vi "CO2_switch_analysis.vi"() -> ()   [LabVIEW 2012]
uses:
  <vilib>/Analysis/3filter.llb/Filter Passband Type.ctl
  <vilib>/Utility/file.llb/Read From Spreadsheet File (DBL).vi
  <vilib>/Analysis/3filter.llb/Zero Phase Filter (DBL).vi
  <vilib>/Utility/file.llb/Write To Spreadsheet File (DBL).vi
  <vilib>/Analysis/NI_AALBase.lvlib
  <vilib>/gmath/NI_Gmath.lvlib
panel:
  out "XY Graph 5":cluster{"Value":dbl[], dbl[]}[](graph)
  in  "Gauss?":bool
  in  "Gauss width scale":dbl(slide) scale=0.0..5.0
  out "Pointer Frame":i32
  out "Point Time":dbl
  in  "Horizontal plot range 3":i32(slide)=564 scale=415.36414565826334..795.514205682273
  out "Analysis Time":dbl
  in  "Multiply SD in Lock-in?":bool
  in  "Average Window":i32(slide)=20 scale=0.0..20.0
  in  "Horizontal plot range 2":cluster{i32, i32, i32, dbl}(slide)={529, 548, 526, 593.2768414505381} scale=403.8640519766044..784.014195885828
  in  "Square Lock-in?":bool
  out "XY Graph 4":cluster{"all rows":dbl[], "all rows":dbl[]}[](graph)
  in  "Lock-in phase":dbl(slide)=2.317171717171717 scale=0.0..6.2
  in  "Lock-in sine Period":dbl(slide)=20.0 step=0.001 scale=19.9..20.1
  out "XY Graph 3":cluster{"Value":dbl[], "Value":dbl[]}[](graph)
  in  "High Pass Filter?":bool=TRUE
  out "1/x":dbl=0.4001580462202354
  in  "Filter order":i32=2
  in  "lowpass":dbl(slide)=0.01 scale=0.0..0.02
  out "Output":dbl[][](array[numeric])
  in  "Write Data":bool
  out "ESCRT":dbl[](array[numeric])
  in  "Horizontal plot range":cluster{i32, i32}(slide)={1038, 1988} scale=0.0..4250.0
  in  "Window":i32(slide)=24 scale=0.0..100.0
  in  "Plot":bool
  in  "Load Data":bool
  out "Data":dbl[][](array[numeric]) format="%0.3f"
  in  "file path (dialog if empty)":path
  in  "stop":bool=TRUE
  out "XY Graph 2":cluster{"Value":dbl[], "Value":dbl[]}[](graph)
  out "XY Graph":cluster{"all rows":dbl[], "all rows":dbl[]}[](graph)
  in  "ESCRT amplitude":i32=22
  in  "Gag Amplitude":i32=12
  in  "Time":i32=3
  out "Time":dbl[](array[numeric])
  # "This program is used to analyze CO2 dependent oscilaltions to determine scission moment. Puncta amplitudes are input as spreedsheet and filtered\nwith lock-in technique using reference that is same frequency as CO2 modulation frequency. The lock-in signal is used to determine scission time. \nTiming of ESCRT recruitment is also determined from amplitude of ESCRT signal."
  # "Array Index"
  # "Column 22. ESCRT Avg Intensity"
  # "Column 23. ESCRT Intensity SD"
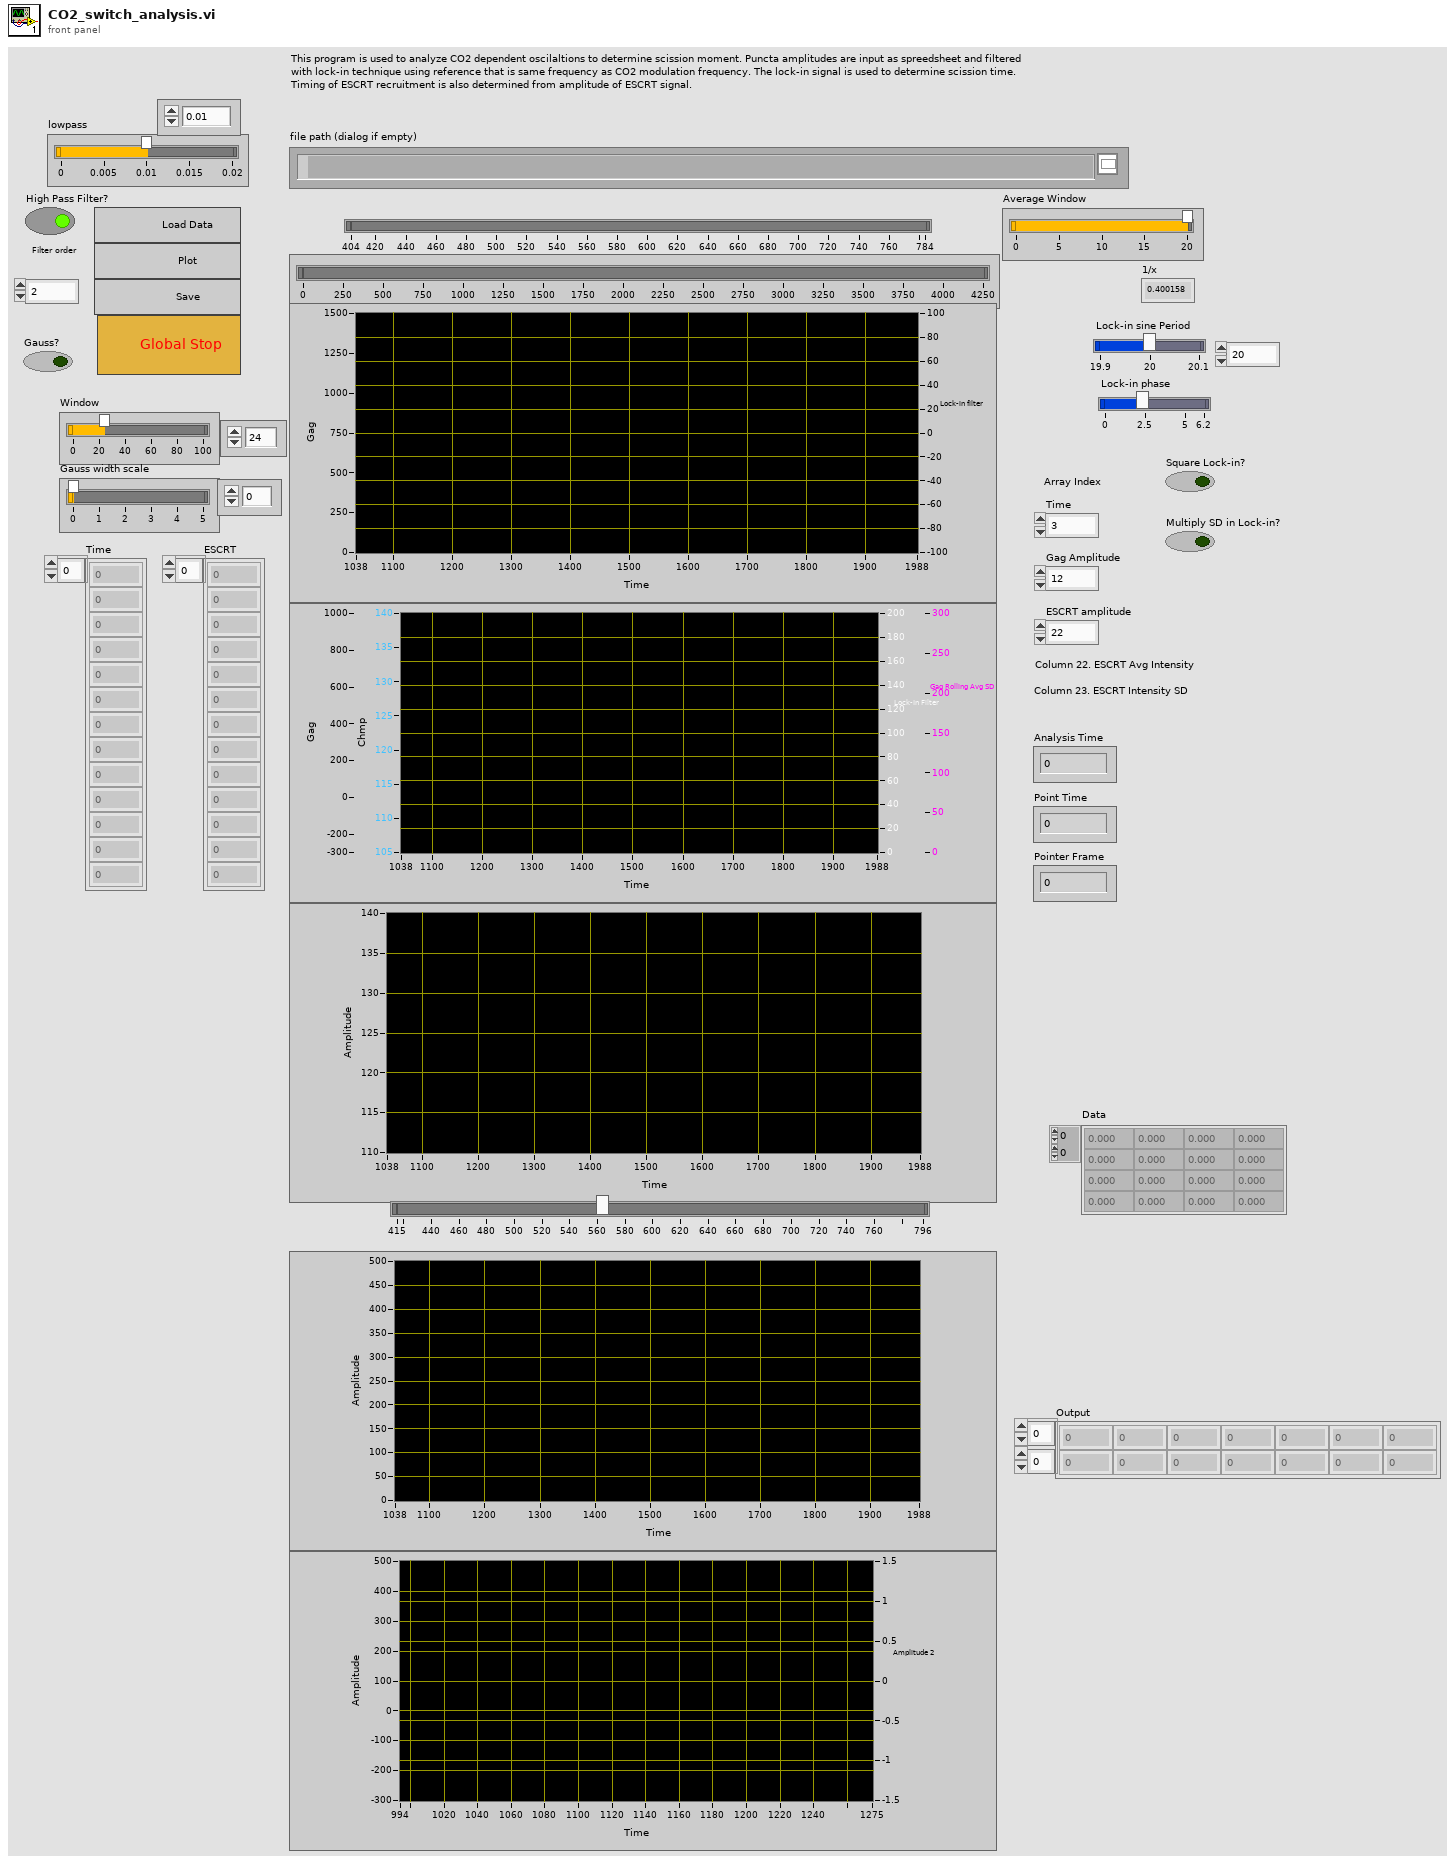
[diagram p1: front panel]
types:
  T1 = typedef "NI_AALBase.lvlib/Filter Passband Type.ctl" = enum32{"Lowpass", "Highpass", "Bandpass", "Bandstop"}
  T2 = cluster{"filter structure":enum32{"IIR 2nd Order", "IIR 4th Order"}, "Reverse Coefficients":dbl[], "Forward Coefficients":dbl[]}
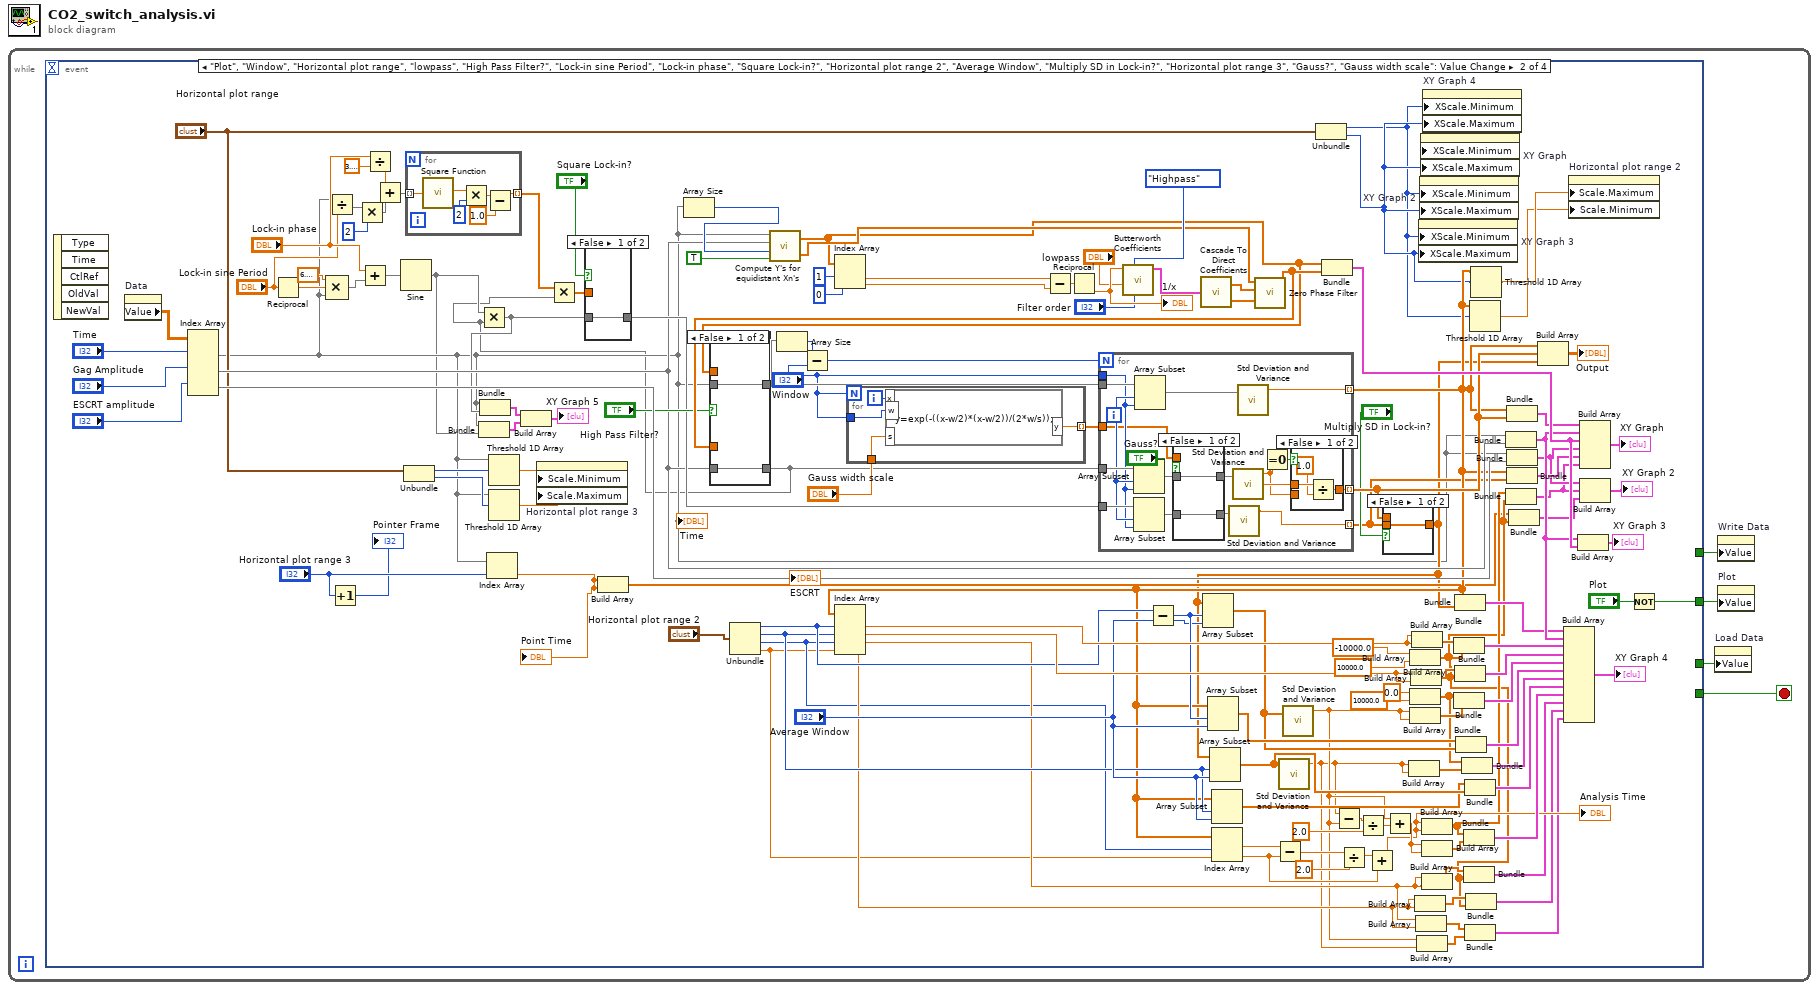
[diagram p0: block diagram]
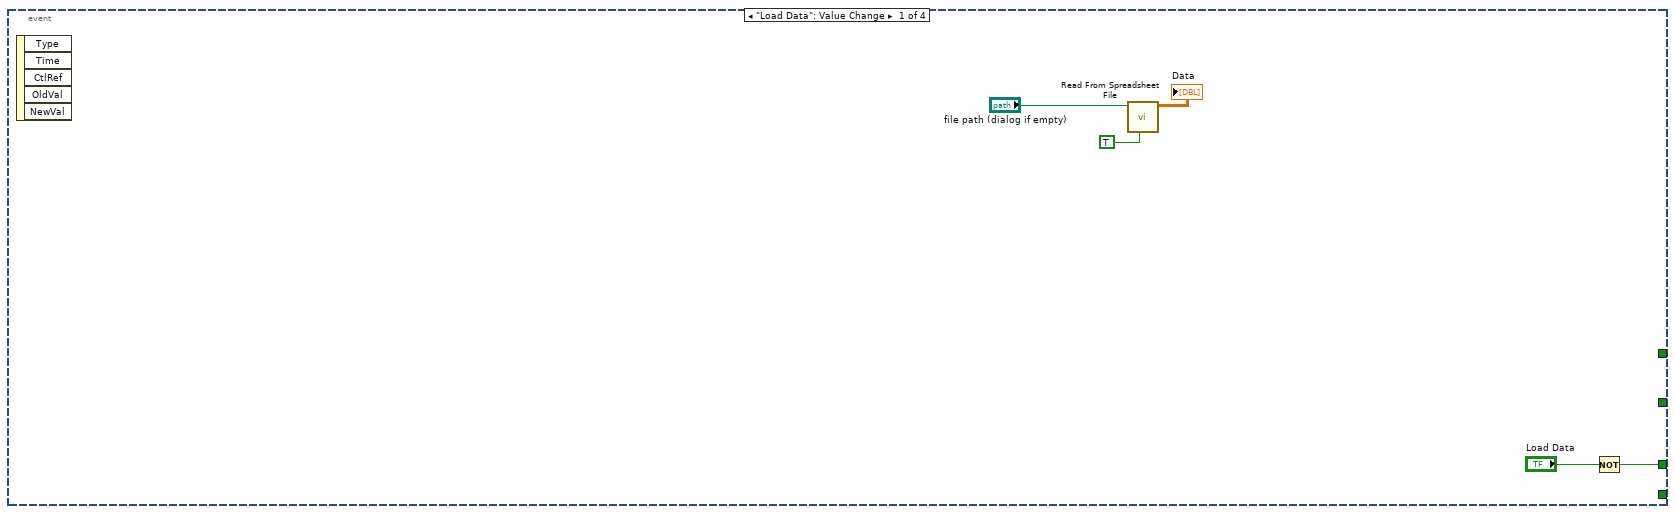
[diagram p2: hidden frame]
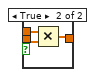
[diagram p3: hidden frame]
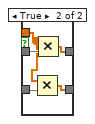
[diagram p6: hidden frame]
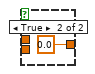
[diagram p7: hidden frame]
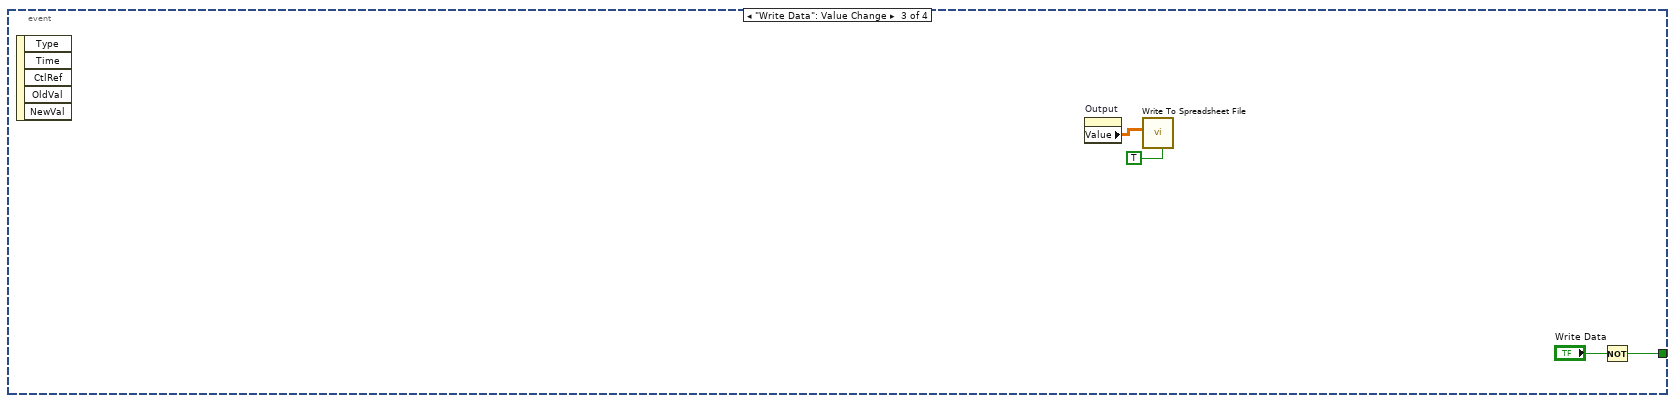
[diagram p8: hidden frame]
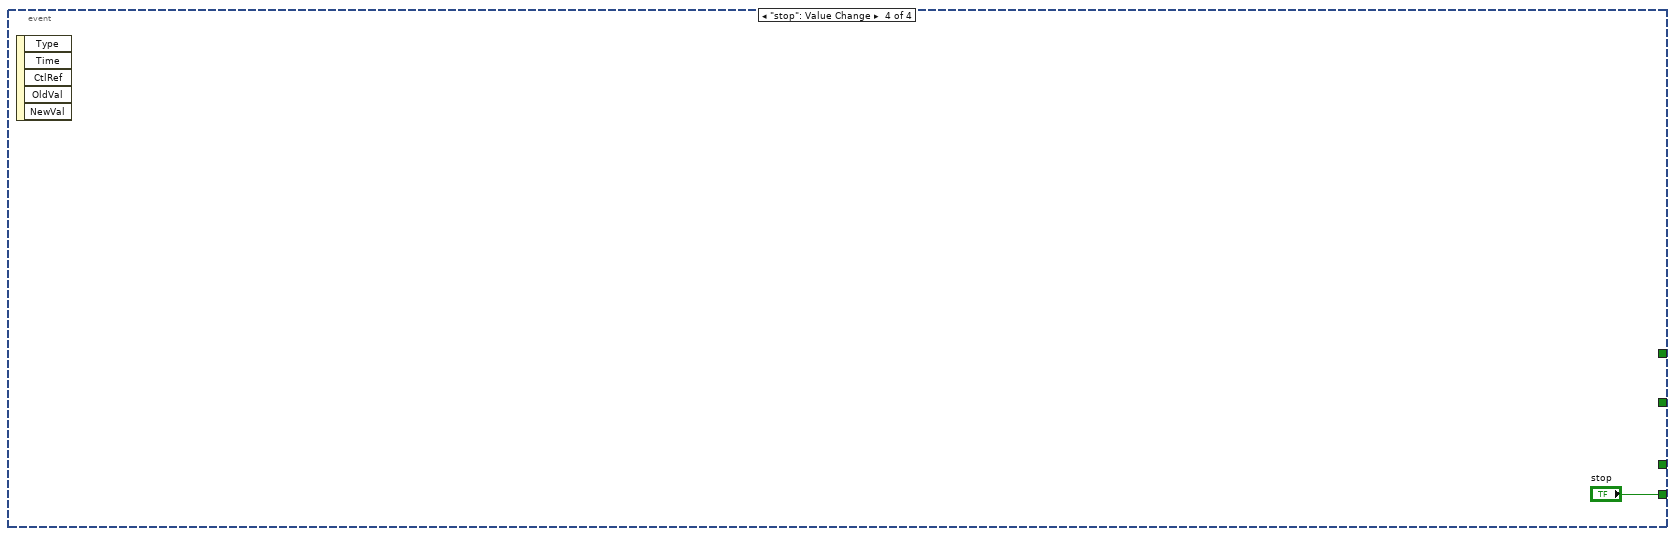
[diagram p9: hidden frame]
diagram:
  n1 = while {
    stop <- w4 stop-if-true
    n2 = event shown="[1] \"Plot\", \"Window\", \"Horizontal plot range\", \"lowpass\", \"High Pass Filter?\", \"Lock-in sine Period\", \"Lock-in phase\", \"Square Lock-in?\", \"Horizontal plot range 2\", \"Average Window\", \"Multiply SD in Lock-in?\", \"Horizontal plot range 3\", \"Gauss?\", \"Gauss width scale\": Value Change" {
      selector: _ -> [_ _ _ _]
      dyn-events: _ -> [_ _ _ _]
      timeout: _ -> [_ _ _ _]
      tunnel: [_ _ _ "stop"] -> w4
      tunnel: [w5 _ _ _] -> w3
      tunnel: [_ w147 _ _] -> w2
      tunnel: [_ _ w200 _] -> w1
      event "Load Data": Value Change {
        n3 = event-data() -> ()  [unwired: 1 in, 5 out]
        n4 = call-poly <vilib>:"Read From Spreadsheet File.vi"("transpose (no:F)"=TRUE, "file path (dialog if empty)"="file path (dialog if empty)") -> ("all rows"=→"Data":dbl[][])  [unwired: 5 in, 4 out]
        n5 = Not(x="Load Data") -> (.not. x?=w5:bool)
      }
      event "Plot", "Window", "Horizontal plot range", "lowpass", "High Pass Filter?", "Lock-in sine Period", "Lock-in phase", "Square Lock-in?", "Horizontal plot range 2", "Average Window", "Multiply SD in Lock-in?", "Horizontal plot range 3", "Gauss?", "Gauss width scale": Value Change {
        n6 = event-data() -> ()  [unwired: 1 in, 5 out]
        n7 = property on="Data" class="Arr (strict)"() -> ("Value"=w142:dbl[][])  [unwired: 2 in, 2 out]
        n8 = Index Array(array=w142, index (row) #1="Time", index (row) #2="Gag Amplitude", index (row) #3="ESCRT amplitude") -> (element #1=w15:dbl[], element #2=w90:dbl[], element #3=w141:dbl[])  [unwired: 3 in]
        "Time" <- w15
        "ESCRT" <- w141
        n9 = Reciprocal(x="Lock-in sine Period") -> (1/x=w116:dbl)
        n10 = Compound Arithmetic op=MULTIPLY(6.283185307179586, w116, w15) -> (w115:dbl[])
        n11 = Divide(x=w15, y="Lock-in sine Period") -> (x/y=w100:dbl[])
        n12 = Increment(x="Horizontal plot range 3") -> (x+1=→"Pointer Frame":i32)
        n13 = Multiply(x=w100, y=2) -> (x*y=w98:dbl[])
        n14 = Add(x="Lock-in phase", y=w115) -> (x+y=w114:dbl[])
        n15 = Divide(x="Lock-in phase", y=3.141592653589793) -> (x/y=w107:dbl)
        n16 = Add(x=w107, y=w98) -> (x+y=w106:dbl[])
        n17 = Sine(x=w114) -> (sin(x)=w14:dbl[])
        n18 = Unbundle("Horizontal plot range") -> (w30:i32, w29:i32)
        n19 = for {
          tunnel: w106 -> [w164] mode=indexing
          tunnel: [w160] -> w102 mode=indexing
          n20 = call <vilib>:"Square Function.vi"("x"=w164) -> ("square(x)"=w163:dbl)
          n21 = Multiply(x=w163, y=2) -> (x*y=w161:dbl)
          n22 = Subtract(x=w161, y=1.0) -> (x-y=w160:dbl)
        }
        n23 = Bundle("Value"=w15, w14) -> (w12:cluster{"Value":dbl[], dbl[]})  [unwired: 1 in]
        n24 = Index Array(array=w15, index="Horizontal plot range 3") -> (element=w31:dbl)
        "Point Time" <- w31
        n25 = Threshold 1D Array(2:w30, 3:w15) -> (0:w25:dbl)  [unwired: 1 in]
        n26 = Threshold 1D Array(2:w29, 3:w15) -> (0:w24:dbl)  [unwired: 1 in]
        n27 = property on="Horizontal plot range 3" class="Slide (strict)"("Scale.Minimum"=w25, "Scale.Maximum"=w24) -> ()  [unwired: 2 in, 2 out]
        n28 = Build Array(w31, w31) -> (w32:dbl[])
        n29 = Array Size(array=w15) -> (size(s)=w120:i32)
        n30 = Unbundle("Horizontal plot range 2") -> (w73:i32, w72:i32, w39:i32, w38:dbl)
        n31 = call "Compute Y's for equidistant Xn's.vi"("Spline(T)"=TRUE, "N"=w120, "Y"=w90, "X"=w15) -> ("Yequi"=w126:dbl[], "Xequi"=w124:dbl[])
        n32 = Index Array(array=w124, index #1=1 ("index"), index #2=0 ("index")) -> (element #1=w136:dbl, element #2=w135:dbl)
        n33 = for {
          N: "Window" -> [_]
          tunnel: "Window" -> [w151]
          tunnel: "Gauss width scale" -> [w150]
          tunnel: [w149] -> w18 mode=indexing
          i -> [w152]
          n34 = formula code="y=exp(-((x-w/2)*(x-w/2))/(2*w/s));"("x"=w152, "w"=w151, "s"=w150) -> ("y"=w149:dbl)
        }
        n35 = Subtract(x=w136, y=w135) -> (x-y=w134:dbl)
        n36 = Reciprocal(x=w134) -> (1/x=w133:dbl)
        "1/x" <- w133
        n37 = call <vilib>:"Butterworth Coefficients.vi"("order"="Filter order", "filter type"=Filter_Passband_Type."Highpass", "low cutoff freq: fl"="lowpass", "sampling freq: fs"=w133) -> ("IIR Filter Cluster"=w129:T2)  [unwired: 6 in, 1 out]
        n38 = Subtract(x=w73, y="Average Window") -> (x-y=w84:i32)
        n39 = call <vilib>:"Cascade To Direct Coefficients.vi"("IIR Filter Cluster"=w129) -> ("Reverse Coefficients"=w128:dbl[], "Forward Coefficients"=w127:dbl[])
        n40 = call-poly <vilib>:"Zero Phase Filter.vi"("Forward Coefficients"=w127, "Reverse Coefficients"=w128, "X"=w126) -> ("Filtered X"=w125:dbl[])  [unwired: 7 in, 1 out]
        n41 = case shown="False" "High Pass Filter?" {
          tunnel: [w166 w168] -> w10
          tunnel: w90 -> [w166 _]
          tunnel: [w165 w167] -> w122
          tunnel: w15 -> [w165 _]
          tunnel: w125 -> [_ w168]
          tunnel: w124 -> [_ w167]
          frame False {
          }
          frame True {
          }
        }
        n42 = Multiply(x=w14, y=w10) -> (x*y=w16:dbl[])
        n43 = Bundle("Value"=w15, w16) -> (w13:cluster{"Value":dbl[], dbl[]})  [unwired: 1 in]
        n44 = Build Array(w13, w12) -> (→"XY Graph 5":cluster{"Value":dbl[], dbl[]}[])
        n45 = Multiply(x=w102, y=w10) -> (x*y=w105:dbl[])
        n46 = case shown="False" "Square Lock-in?" {
          tunnel: w16 -> [w157 _]
          tunnel: [w157 w158] -> w103
          tunnel: w105 -> [_ w158]
          frame False {
          }
          frame True {
          }
        }
        n47 = Array Size(array=w122) -> (size(s)=w123:i32)
        n48 = Subtract(x=w123, y="Window") -> (x-y=w20:i32)
        n49 = for {
          N: w20 -> [_]
          tunnel: w122 -> [w186]
          tunnel: "Window" -> [w176]
          tunnel: [w184] -> w59 mode=indexing
          tunnel: w10 -> [w183]
          tunnel: [w180] -> w61 mode=indexing
          tunnel: [w169] -> w58 mode=indexing
          tunnel: w103 -> [w178]
          tunnel: w18 -> [w173]
          i -> [w177]
          n50 = Array Subset(array=w183, index=w177, length=w176) -> (w175:dbl[])
          n51 = Array Subset(array=w178, index=w177, length=w176) -> (w171:dbl[])
          n52 = Array Subset(array=w186, index=w177, length=w176) -> (w185:dbl[])
          n53 = case shown="False" "Gauss?" {
            tunnel: w175 -> [w188 w193]
            tunnel: [w188 w192] -> w174
            tunnel: w173 -> [_ w189]
            tunnel: w171 -> [w187 w190]
            tunnel: [w187 w191] -> w170
            frame False {
            }
            frame True {
              n54 = Multiply(x=w189, y=w190) -> (x*y=w191:dbl[])
              n55 = Multiply(x=w189, y=w193) -> (x*y=w192:dbl[])
            }
          }
          n56 = call <vilib>:"Std Deviation and Variance.vi"("X"=w170) -> ("mean"=w169:dbl)  [unwired: 1 in, 2 out]
          n57 = call <vilib>:"Std Deviation and Variance.vi"("X"=w174) -> ("mean"=w179:dbl, "standard deviation"=w181:dbl)  [unwired: 1 in, 1 out]
          n58 = call <vilib>:"Std Deviation and Variance.vi"("X"=w185) -> ("mean"=w184:dbl)  [unwired: 1 in, 2 out]
          n59 = Equal To 0?(x=w179) -> (x = 0?=w182:bool)
          n60 = case shown="False" w182 {
            tunnel: w179 -> [_ _]
            tunnel: w181 -> [w196 _]
            tunnel: [w195 0.0] -> w180
            frame False {
              n61 = Divide(x=w196, y=1.0) -> (x/y=w195:dbl)
            }
            frame True {
            }
          }
        }
        n62 = Index Array(array=w59, index #1=w73, index #2=w72, index #3=w39, index #4=w38) -> (element #1=w89:dbl, element #2=w93:dbl, element #3=w47:dbl, element #4=w46:dbl)
        n63 = Array Subset(array=w59, index=w84, length="Average Window") -> (w83:dbl[])
        n64 = Array Subset(array=w59, index=w72, length="Average Window") -> (w76:dbl[])
        n65 = Index Array(array=w59, index #1=w39, index #2=w38) -> (element #1=w66:dbl, element #2=w62:dbl)
        n66 = Subtract(x=w66, y=w62) -> (x-y=w65:dbl)
        n67 = Unbundle("Horizontal plot range") -> (w35:i32, w36:i32)
        n68 = Bundle("Xequi"=w124, "Filtered X"=w125) -> (w118:cluster{"Xequi":dbl[], "Filtered X":dbl[]})  [unwired: 1 in]
        n69 = Divide(x=w65, y=2.0) -> (x/y=w63:dbl)
        n70 = Add(x=w63, y=w62) -> (x+y=w56:dbl)
        "Analysis Time" <- w56
        n71 = case shown="False" "Multiply SD in Lock-in?" {
          tunnel: w58 -> [w153 w155]
          tunnel: [w153 w156] -> w21
          tunnel: w61 -> [_ w154]
          frame False {
          }
          frame True {
            n72 = Multiply(x=w154, y=w155) -> (x*y=w156:dbl[])
          }
        }
        n73 = Array Subset(array=w21, index=w84, length="Average Window") -> (w82:dbl[])
        n74 = Array Subset(array=w21, index=w72, length="Average Window") -> (w77:dbl[])
        n75 = call <vilib>:"Std Deviation and Variance.vi"("X"=w77) -> ("mean"=w44:dbl)  [unwired: 1 in, 2 out]
        n76 = call <vilib>:"Std Deviation and Variance.vi"("X"=w82) -> ("mean"=w45:dbl)  [unwired: 1 in, 2 out]
        n77 = Subtract(x=w44, y=w45) -> (x-y=w70:dbl)
        n78 = Divide(x=w70, y=2.0) -> (x/y=w68:dbl)
        n79 = Add(x=w45, y=w68) -> (x+y=w67:dbl)
        n80 = Build Array(w44, w44) -> (w79:dbl[])
        n81 = Build Array(-10000.0 ("element"), 10000.0 ("element")) -> (w33:dbl[])
        n82 = Build Array(0.0 ("element"), 10000.0 ("element")) -> (w80:dbl[])
        n83 = Build Array(w45, w45) -> (w86:dbl[])
        n84 = Build Array(w93, w93) -> (w92:dbl[])
        n85 = Build Array(w89, w89) -> (w96:dbl[])
        n86 = Build Array(w46, w46) -> (w49:dbl[])
        n87 = Build Array(w47, w46) -> (w42:dbl[])
        n88 = Build Array(w45, w44) -> (w43:dbl[])
        n89 = property on="XY Graph 3" class="XYGraph (strict)"("XScale.Minimum"=w35, "XScale.Maximum"=w36) -> ()  [unwired: 2 in, 2 out]
        n90 = property on="XY Graph 2" class="XYGraph (strict)"("XScale.Minimum"=w35, "XScale.Maximum"=w36) -> ()  [unwired: 2 in, 2 out]
        n91 = property on="XY Graph" class="XYGraph (strict)"("XScale.Minimum"=w35, "XScale.Maximum"=w36) -> ()  [unwired: 2 in, 2 out]
        n92 = Build Array(w56, w56) -> (w52:dbl[])
        n93 = Build Array(w67, w67) -> (w53:dbl[])
        n94 = Build Array(w47, w47) -> (w50:dbl[])
        n95 = property on="XY Graph 4" class="XYGraph (strict)"("XScale.Minimum"=w35, "XScale.Maximum"=w36) -> ()  [unwired: 2 in, 2 out]
        n96 = Bundle(w96, w33) -> (w97:cluster{dbl[], dbl[]})  [unwired: 1 in]
        n97 = Bundle(w80, w86) -> (w85:cluster{dbl[], dbl[]})  [unwired: 1 in]
        n98 = Bundle(w59, w21) -> (w110:cluster{dbl[], dbl[]})  [unwired: 1 in]
        n99 = Bundle(w92, w33) -> (w91:cluster{dbl[], dbl[]})  [unwired: 1 in]
        n100 = Bundle(w83, w82) -> (w81:cluster{dbl[], dbl[]})  [unwired: 1 in]
        n101 = Bundle(w80, w79) -> (w78:cluster{dbl[], dbl[]})  [unwired: 1 in]
        n102 = Bundle(w52, w53) -> (w71:cluster{dbl[], dbl[]})  [unwired: 1 in]
        n103 = Bundle(w50, w33) -> (w51:cluster{dbl[], dbl[]})  [unwired: 1 in]
        n104 = Bundle(w76, w77) -> (w75:cluster{dbl[], dbl[]})  [unwired: 1 in]
        n105 = Bundle(w42, w43) -> (w41:cluster{dbl[], dbl[]})  [unwired: 1 in]
        n106 = Bundle(w49, w33) -> (w48:cluster{dbl[], dbl[]})  [unwired: 1 in]
        n107 = Threshold 1D Array(2:w35, 3:w59) -> (0:w26:dbl)  [unwired: 1 in]
        n108 = Threshold 1D Array(2:w36, 3:w59) -> (0:w27:dbl)  [unwired: 1 in]
        n109 = Bundle("Value"=w15, "Value"=w90) -> (w111:cluster{"Value":dbl[], "Value":dbl[]})  [unwired: 1 in]
        n110 = Bundle(w52, w33) -> (w37:cluster{dbl[], dbl[]})  [unwired: 1 in]
        n111 = Bundle(w59, w61) -> (w112:cluster{dbl[], dbl[]})  [unwired: 1 in]
        n112 = Bundle("Value"=w15, "Value"=w141) -> (w55:cluster{"Value":dbl[], "Value":dbl[]})  [unwired: 1 in]
        n113 = Bundle(w59, w58) -> (w57:cluster{dbl[], dbl[]})  [unwired: 1 in]
        n114 = Bundle(w32, w33) -> (w34:cluster{dbl[], dbl[]})  [unwired: 1 in]
        n115 = Build Array(w59, w61, w21) -> (→"Output":dbl[][])
        n116 = Build Array(w110, w111, w97, w91, w85, w81, w78, w75, w71, w51, w48, w41) -> (→"XY Graph 4":cluster{"Value":dbl[], "Value":dbl[]}[])
        n117 = property on="Horizontal plot range 2" class="Slide (strict)"("Scale.Maximum"=w27, "Scale.Minimum"=w26) -> ()  [unwired: 2 in, 2 out]
        n118 = Build Array(w111, w118) -> (→"XY Graph 3":cluster{"Xequi":dbl[], "Filtered X":dbl[]}[])
        n119 = Build Array(w112, w111, w118, w55, w57, w37) -> (→"XY Graph":cluster{"Value":dbl[], "Value":dbl[]}[])
        n120 = Build Array(w55, w37, w34) -> (→"XY Graph 2":cluster{"Value":dbl[], "Value":dbl[]}[])
        n121 = Not(x="Plot") -> (.not. x?=w147:bool)
      }
      event "Write Data": Value Change {
        n122 = event-data() -> ()  [unwired: 1 in, 5 out]
        n123 = property on="Output" class="Arr (strict)"() -> ("Value"=w199:dbl[][])  [unwired: 2 in, 2 out]
        n124 = call-poly <vilib>:"Write To Spreadsheet File.vi"("transpose? (no:F)"=TRUE, "2D data"=w199) -> ()  [unwired: 6 in, 1 out]
        n125 = Not(x="Write Data") -> (.not. x?=w200:bool)
      }
      event "stop": Value Change {
        n126 = event-data() -> ()  [unwired: 1 in, 5 out]
      }
    }
    n127 = property on="Load Data" class="Bool (strict)"("Value"=w3) -> ()  [unwired: 2 in, 2 out]
    n128 = property on="Write Data" class="Bool (strict)"("Value"=w1) -> ()  [unwired: 2 in, 2 out]
    n129 = property on="Plot" class="Bool (strict)"("Value"=w2) -> ()  [unwired: 2 in, 2 out]
  }
